vi "Get Bit Depth.vi"(8 "error in (no error)":errorcluster, 10 "depth":i32, 11 "channel":i32) -> (0 "error out":errorcluster, 2 "depth out":i32, 3 "function return":u32)   [LabVIEW 2014, in "atmcd32d.lvlib"]
doc: "unsigned int WINAPI GetBitDepth(int channel, int * depth);"
uses:
  atmcd32d.lvlib
  atmcd32d.dll
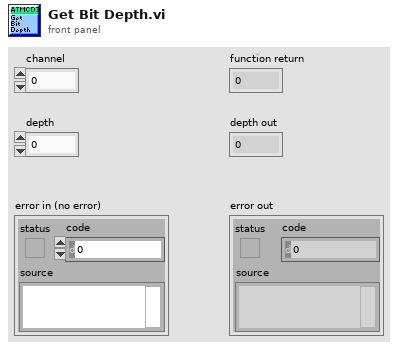
[diagram p1: front panel]
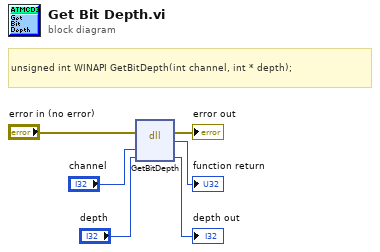
[diagram p0: block diagram]
diagram:
  # "unsigned int WINAPI GetBitDepth(int channel, int * depth);"
  n1 = dll-call lib="C:/Users/Bakir/Documents/Lambda2-Testing/lib/Andorlib/atmcd32d.*" fn="GetBitDepth"(error in="error in (no error)", "channel"="channel", "depth"="depth") -> (error out=→"error out":errorcluster, →"function return":u32, "depth"=→"depth out":i32)  [unwired: 3 in, 1 out]
